vi "Insert Stop Loop.vi"(8 "error in (no error)":errorcluster, 10 "Insert Stop Loop":T1, 11 "Test Executive Builder in":refnum<class "Test Executive Builder.lvclass">) -> (0 "error out":errorcluster, 3 "Test Executive Builder out":refnum<class "Test Executive Builder.lvclass">, 5 "Unique ID out":string)   [LabVIEW 2017, in "Test Executive Builder.lvclass"]
uses:
  Test Executive Builder.lvclass
  Source/Test Executive Builder Model/Test Executive Builder Model/Test Executive Builder Model.lvclass
  d5f03b32-5504-413a-ab36-7bacdf6bb31a.vi
  C:/Users/jonmc/Documents/Git/Test Executive Builder/Source/Test Executive Builder Model/Test Executive Builder Model/Test Executive Builder Model.lvclass
  Source/Test Executive Builder Dialogs/ITest Executive Builder Dialog/ITest Executive Builder Dialog.lvclass
  Source/Application Dependencies/Insert Stop Loop.ctl
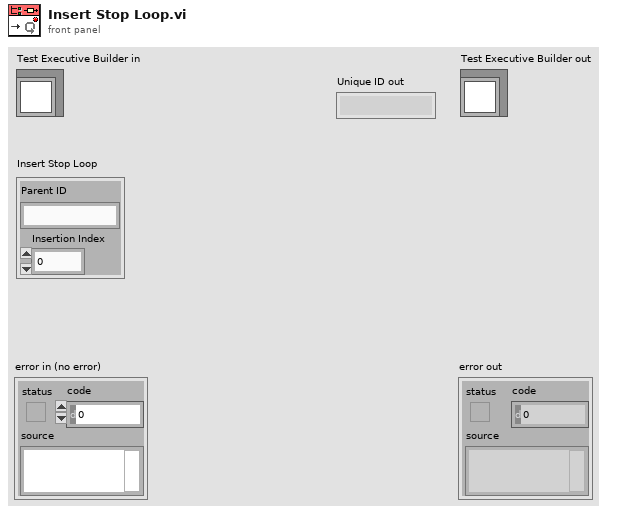
[diagram p1: front panel]
types:
  T1 = typedef "Insert Stop Loop.ctl" = cluster{"Parent ID":string, "Insertion Index":i32}
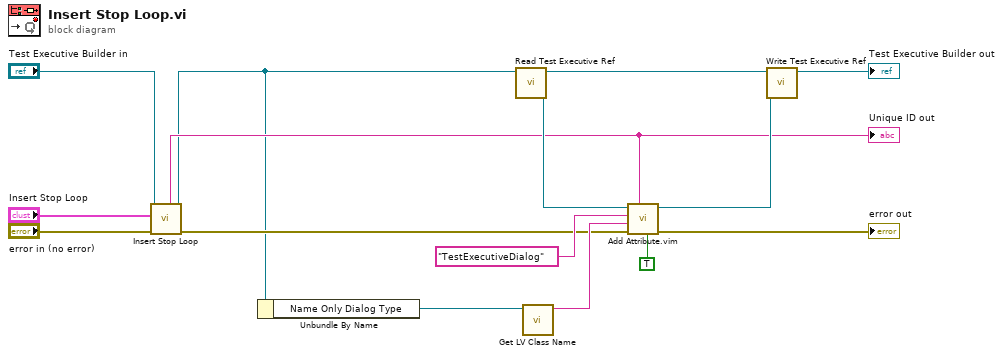
[diagram p0: block diagram]
diagram:
  n1 = call-parent "Insert Stop Loop.vi"("error in (no error)"="error in (no error)", "Insert Stop Loop"="Insert Stop Loop", "Test Executive Builder Model in"="Test Executive Builder in") -> ("error out"=w4:errorcluster, "Test Executive Builder Model out"=w2:refnum<class "Test Executive Builder.lvclass">, "Unique ID out"=w5:string)  [unwired: 6 in]
  "Unique ID out" <- w5
  n2 = Unbundle By Name(w2) -> ("Name Only Dialog Type"=w1:refnum<class "ITest Executive Builder Dialog.lvclass">)
  n3 = call "Read Test Executive Ref.vi"("Test Executive Builder Model in"=w2) -> ("Test Executive Ref"=w11:refnum<data-value>, "Test Executive Builder Model out"=w12:refnum<class "Test Executive Builder.lvclass">)  [unwired: 9 in]
  n4 = call <vilib>:"Get LV Class Name.vi"("object"=w1) -> ("class name"=w7:string)  [unwired: 9 in, 1 out]
  n5 = call "Add Attribute.vim"("Private?"=TRUE, "ID"=w5, "error in (no error)"=w4, "Attribute"=w7, "Attribute Name"="TestExecutiveDialog", "Test Executive Ref"=w11) -> ("error out"=→"error out":errorcluster, "Test Executive Ref out"=w10:refnum<data-value>)  [unwired: 2 in, 2 out]
  n6 = call "Write Test Executive Ref.vi"("Test Executive Ref"=w10, "Test Executive Builder Model in"=w12) -> ("Test Executive Builder Model out"=→"Test Executive Builder out":refnum<class "Test Executive Builder.lvclass">)  [unwired: 9 in]
